vi "FLiNaK Density.vi"(11 "FLiNaK Temp (K)":dbl) -> (3 "FLiNaK Density (kg/m^3)":dbl)   [LabVIEW 2019]
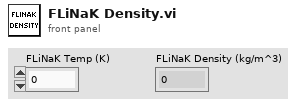
[diagram p1: front panel]
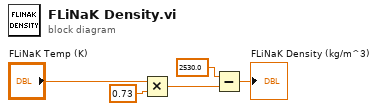
[diagram p0: block diagram]
diagram:
  n1 = Multiply(x="FLiNaK Temp (K)", y=0.73) -> (x*y=w4:dbl)
  n2 = Subtract(x=2530.0, y=w4) -> (x-y=→"FLiNaK Density (kg/m^3)":dbl)
